vi "Config Zone.vi"(0 "VISA resource name":refnum<visa-resource-name>, 1 "Zone (1)":i32=1 min=1 max=10 step=1, 2 "Setpoint Limit (0.00000E+0)":dbl min=0.0 max=100000000.0 step=1e-06 format="%^.5e", 3 "Heater Manual Output (0.000)":dbl min=0.0 max=100.0 step=0.001 format="%.3f", 4 "Analog 1 Output (0.000 %)":dbl min=-100.0 max=100.0 step=0.001 format="%.3f", 5 "Analog 2 Output (0.000 %)":dbl min=-100.0 max=100.0 step=0.001 format="%.3f", 6 "Heater Range (0: Off)":u16(ring) items=["Off", "31.6 uA", "100 uA", "316 uA", "1.00 mA", "3.16 mA", "10.0 mA", "31.6 mA", "100 mA"], 7 "error in (no error)":errorcluster, 8 "Gain(P) (10.000)":dbl=10.0 min=0.001 max=1000.0 step=0.001 format="%.3f", 9 "Relay Low (0: Off)":u16(ring) items=["Off", "On"], 10 "Reset(I) (20)":dbl=20.0 min=0.0 max=10000.0 step=1.0, 11 "Relay High (0: Off)":u16(ring) items=["Off", "On"], 12 "Rate(D) (0)":dbl min=0.0 max=2500.0 step=1.0) -> (20 "VISA resource name out":refnum<visa-resource-name>, 27 "error out":errorcluster)   [LabVIEW 2020, in "Lake Shore Cryotronics 370.lvlib"]
doc: "This VI Configures the parameters of the zone table."
uses:
  Lake Shore Cryotronics 370.lvlib
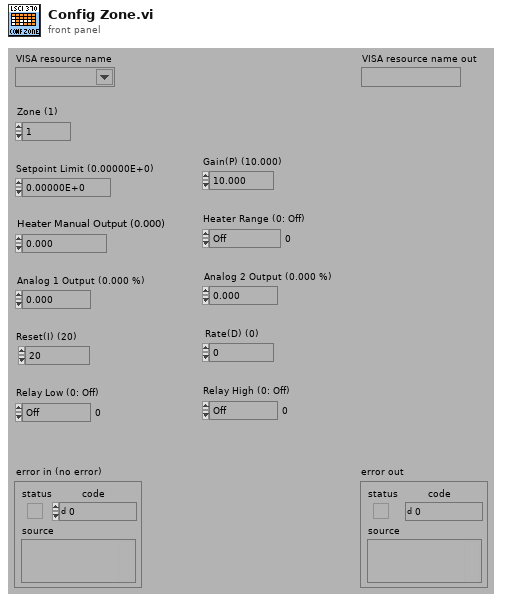
[diagram p1: front panel]
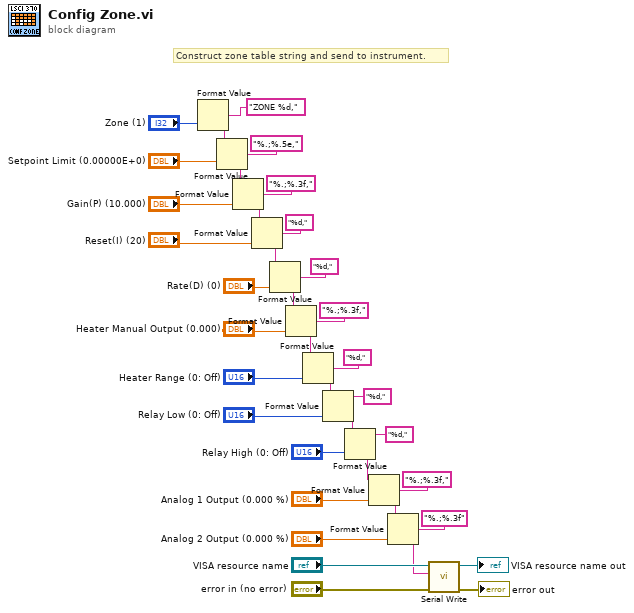
[diagram p0: block diagram]
diagram:
  # "Construct zone table string and send to instrument."
  n1 = Format Value(format string="ZONE %d,", value (0)="Zone (1)") -> (output string=w30:string)  [unwired: 1 in]
  n2 = Format Value(string ("")=w30, format string="%.;%.5e,", value (0)="Setpoint Limit (0.00000E+0)") -> (output string=w19:string)
  n3 = Format Value(string ("")=w19, format string="%.;%.3f,", value (0)="Gain(P) (10.000)") -> (output string=w24:string)
  n4 = Format Value(string ("")=w24, format string="%d,", value (0)="Reset(I) (20)") -> (output string=w23:string)
  n5 = Format Value(string ("")=w23, format string="%d,", value (0)="Rate(D) (0)") -> (output string=w20:string)
  n6 = Format Value(string ("")=w20, format string="%.;%.3f,", value (0)="Heater Manual Output (0.000)") -> (output string=w21:string)
  n7 = Format Value(string ("")=w21, format string="%d,", value (0)="Heater Range (0: Off)") -> (output string=w11:string)
  n8 = Format Value(string ("")=w11, format string="%d,", value (0)="Relay Low (0: Off)") -> (output string=w10:string)
  n9 = Format Value(string ("")=w10, format string="%d,", value (0)="Relay High (0: Off)") -> (output string=w5:string)
  n10 = Format Value(string ("")=w5, format string="%.;%.3f,", value (0)="Analog 1 Output (0.000 %)") -> (output string=w4:string)
  n11 = Format Value(string ("")=w4, format string="%.;%.3f", value (0)="Analog 2 Output (0.000 %)") -> (output string=w3:string)
  n12 = call "Serial Write.vi"("error in (no error)"="error in (no error)", "Write Buffer (\"\")"=w3, "VISA resource name"="VISA resource name") -> ("error out"=→"error out":errorcluster, "VISA resource name out"=→"VISA resource name out":refnum<visa-resource-name>)  [unwired: 6 in, 1 out]
